vi "2RMS9225-7_FPGA.vi"(1 "Amplitude [p.u.]":fxp<+,36,0>) -> (0 "Amplitude [RMS p.u.]":fxp<+,36,0>)   [LabVIEW 2021]
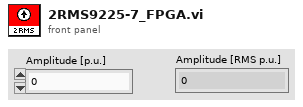
[diagram p1: front panel]
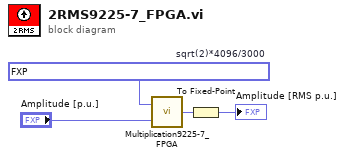
[diagram p0: block diagram]
diagram:
  w4 = fxp<+/-,47,6> 1.9308729171602863  # sqrt(2)*4096/3000
  n1 = call "Multiplication9225-7_FPGA.vi"("y <+/-44,8>"="Amplitude [p.u.]", "x <+/-47,6>"=w4) -> ("x*y <+/-49,13>"=w3:fxp<+/-,49,13>)
  n2 = To Fixed-Point(number=w3) -> (fixed-point=→"Amplitude [RMS p.u.]":fxp<+,36,0>)  [unwired: 1 in]
